vi "USB9825_DO.vi"(8 "Error In":errorcluster caption="错误输入", 10 "pDO":i32=255 format="%x", 11 "hDevice":i32) -> (0 "Error Out":errorcluster caption="错误输出")   [LabVIEW 2015, in "DAQ.lvlib"]
uses:
  DAQ.lvlib
  USB9825.DLL
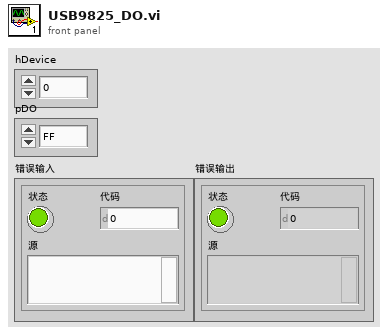
[diagram p1: front panel]
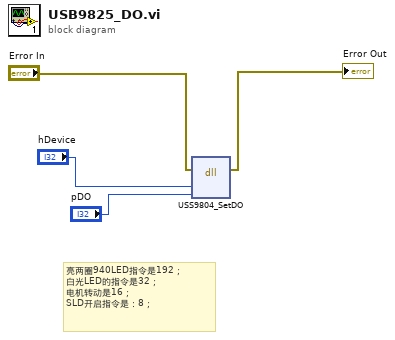
[diagram p0: block diagram]
diagram:
  # "亮两圈940LED指令是192；\n白光LED的指令是32；\n电机转动是16；\nSLD开启指令是：8；"
  n1 = dll-call lib="PTH2sabs CYexinrongWorkplace\t普密斯Thickness-measurementBiometry_alpha3 bolihouduSub VIsDAQUSB9825.dll" fn="USS9804_SetDO"(error in="Error In", "hDevice"="hDevice", "pDO"="pDO") -> (error out=→"Error Out":errorcluster)  [unwired: 5 in, 1 out]
